vi "ST TCP SoundCheck Control - Run Sequence.vi"(8 "error in (no error)":errorcluster, 9 "TimeOut(s)":dbl=60.0, 11 "TCP Cnct in":refnum<k5>) -> (0 "error out":errorcluster, 1 "Duration":dbl, 2 "Success?":bool, 3 "TCP Cnct out":refnum<k5>)   [LabVIEW 2018]
uses:
  <vilib>/KATE/Time/Time Utils.lvlib
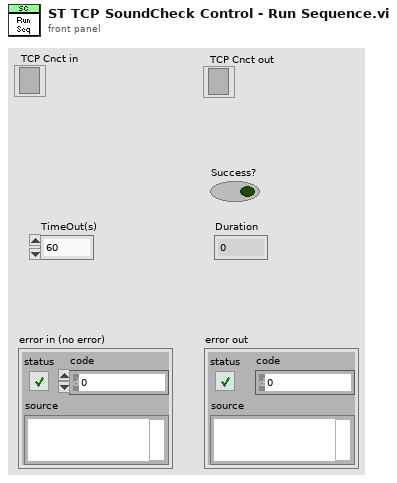
[diagram p1: front panel]
types:
  T1 = typedef "SC TCP SequenceRun.ctl" = cluster{"Success?":bool, "Pass?":bool, "Margin":dbl, "StepResults":T2[]}
  T2 = typedef "SC TCP StepResult.ctl" = cluster{"Evaluated":bool, "Verdict":bool, "Margin":dbl, "Limit":string, "Max/Min":string}
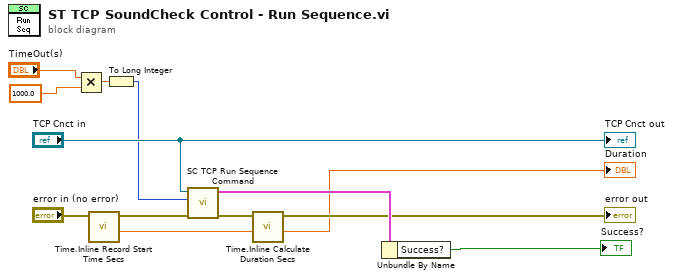
[diagram p0: block diagram]
diagram:
  n1 = Multiply(x="TimeOut(s)", y=1000.0) -> (x*y=w2:dbl)
  n2 = call <vilib>:"Time.Inline Record Start Time Secs.vi"("Error In Upper"="error in (no error)") -> ("Start(s)"=w6:dbl, "Error Out Upper"=w10:errorcluster)  [unwired: 8 in, 1 out]
  n3 = To Long Integer(number=w2) -> (32bit integer=w1:i32)
  n4 = call "SC TCP Run Sequence Command.vi"("error in (no error)"=w10, "timeout (ms)"=w1, "TCP Network Connection in"="TCP Cnct in") -> ("error out"=w8:errorcluster, "Return"=w13:T1)  [unwired: 7 in]
  n5 = call <vilib>:"Time.Inline Calculate Duration Secs.vi"("Start(Sec)"=w6, "Error In Top"=w8) -> ("Duration(s)"=→"Duration":dbl, "Error Out Top"=→"error out":errorcluster)  [unwired: 7 in, 1 out]
  n6 = Unbundle By Name(w13) -> ("Success?"=→"Success?":bool)
  "TCP Cnct out" <- "TCP Cnct in"
